vi "Enqueue (Array).vi"(4 "timeout in ms (-1)":i32=-1, 6 "Priority Message? Array":bool[](array[boolean]), 8 "error in (no error)":errorcluster, 9 "Message Data Array":variant[](array[variant]), 10 "States":T2[](array[typedef]), 11 "Message Queue":T1) -> (0 "error out":errorcluster, 3 "dup Message Queue":T1)   [LabVIEW 2019, in "Message Queue.lvlib"]
doc: "For a regular message, enqueue the message. For a priority message, enqueue it at the front of the queue."
uses:
  Message Queue.lvlib
  State Name.ctl
  Shared/TypeDefs/Message Queue Ref.ctl
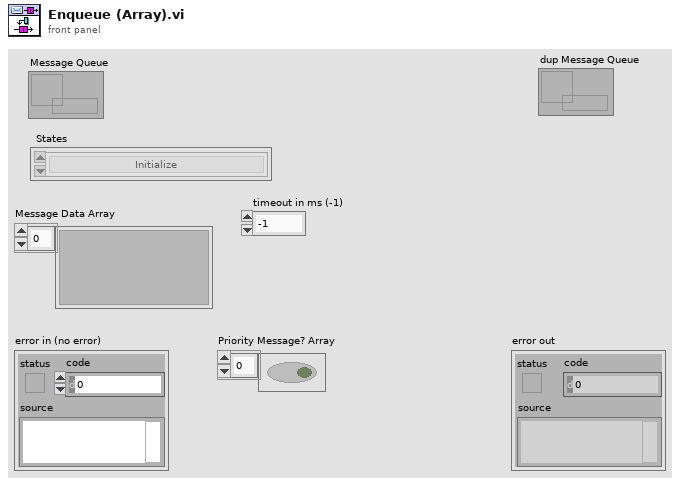
[diagram p1: front panel]
types:
  T1 = typedef "Message Queue Ref.ctl" = refnum<queue>
  T2 = typedef "Message Queue.lvlib/State Name.ctl" = enum16{"Default", "Initialize", "Initialize Data", "Initialize Modules", "Initialize Panel", "Close FP", "Open FP", "Initialize Menu", "Mode", "Update Subpanel", "Error", "Open Help", "About", "Open WebResources", "Exit"}
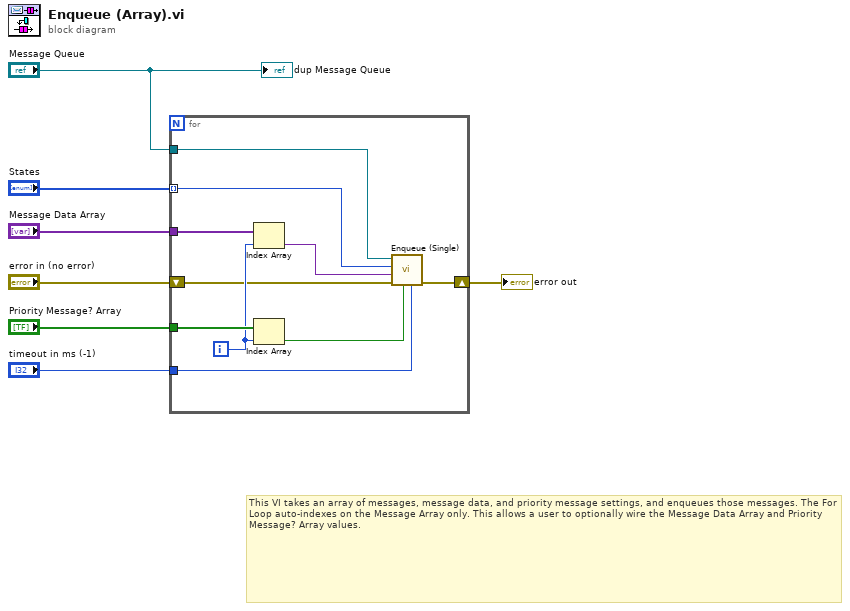
[diagram p0: block diagram]
diagram:
  # "This VI takes an array of messages, message data, and priority message settings, and enqueues those messages. The For Loop auto-indexes on the Message Array only. This allows a user to optionally wire the Message Data Array and Priority Message? Array values."
  n1 = for {
    tunnel: "Message Data Array" -> [w17]
    tunnel: "Priority Message? Array" -> [w16]
    tunnel: "Message Queue" -> [w14]
    shift-right: [w8] -> w4
    shift-left: "error in (no error)" -> [w11]
    tunnel: "States" -> [w13] mode=indexing
    tunnel: "timeout in ms (-1)" -> [w9]
    i -> [w15]
    n2 = Index Array(array=w17, index=w15) -> (element=w12:variant)
    n3 = Index Array(array=w16, index=w15) -> (element=w10:bool)
    n4 = call "Enqueue (Single).vi"("timeout in ms (-1)"=w9, "Priority Message? Array"=w10, "error in (no error)"=w11, "Message Data Array"=w12, "States"=w13, "Message Queue"=w14) -> ("error out"=w8:errorcluster)  [unwired: 4 in, 1 out]
  }
  "error out" <- w4
  "dup Message Queue" <- "Message Queue"
